vi "Track Array Replace.vi"(8 "连接端":enum16{"无连接", "前端", "后端", "前后端"}(ring), 9 "num":i32=1, 11 "output array":string[][](array[string])) -> (3 "output array 2":string[][](array[string]))   [LabVIEW 2015]
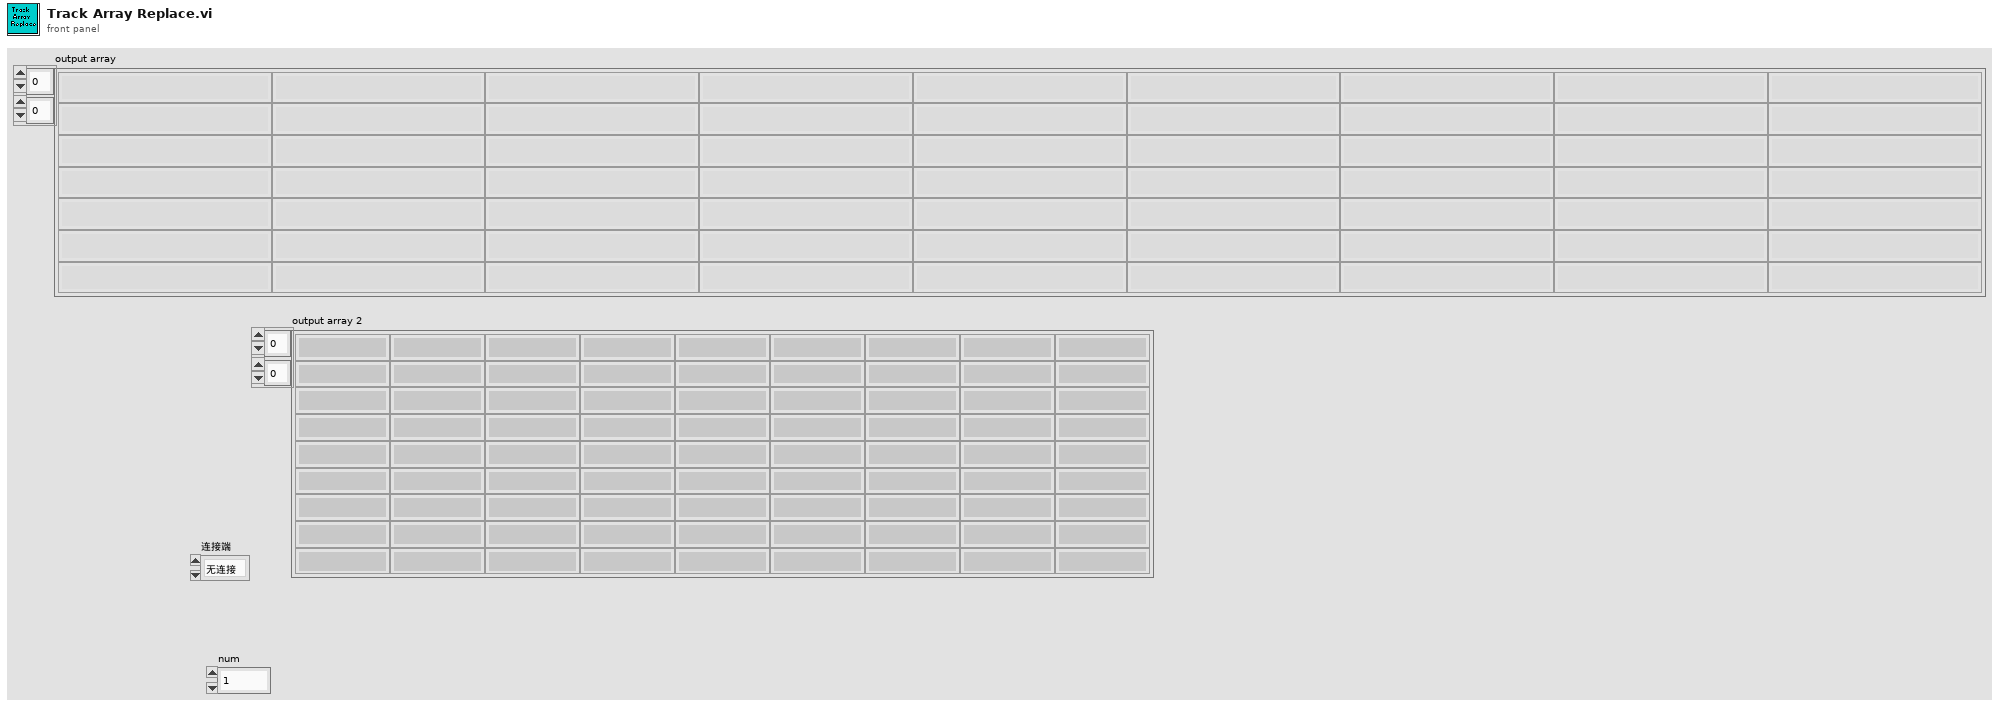
[diagram p1: front panel]
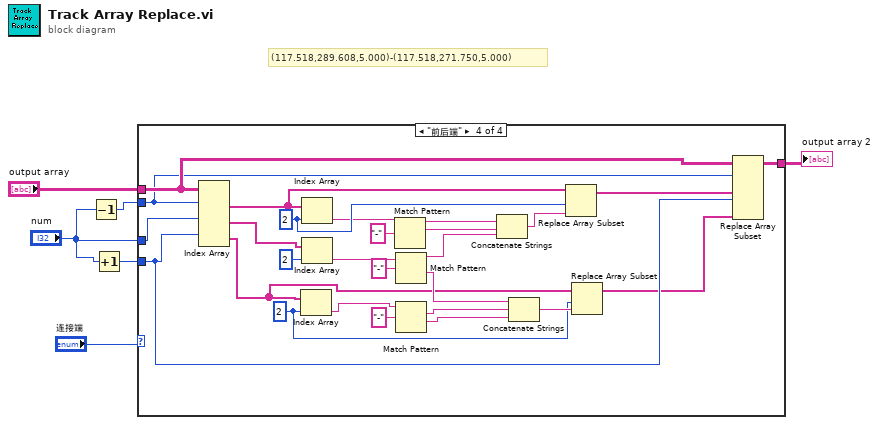
[diagram p0: block diagram]
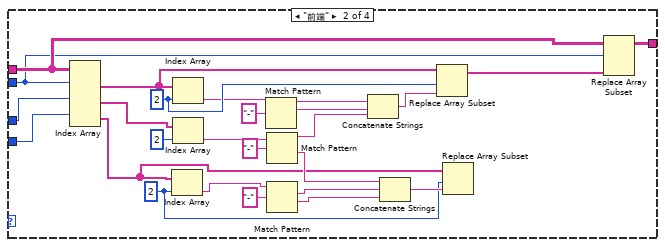
[diagram p3: hidden frame]
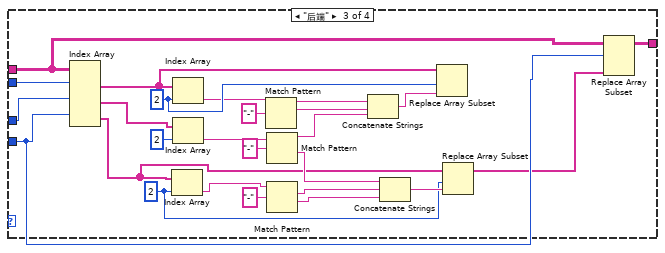
[diagram p4: hidden frame]
diagram:
  # "(117.518,289.608,5.000)-(117.518,271.750,5.000)"
  n1 = Decrement(x="num") -> (x-1=w4:i32)
  n2 = Increment(x="num") -> (x+1=w3:i32)
  n3 = case shown="\"前后端\"" "连接端" {
    tunnel: "num" -> [_ w33 w59 w86]
    tunnel: "output array" -> [w7 w12 w38 w65]
    tunnel: w4 -> [_ w11 w37 w64]
    tunnel: w3 -> [_ w9 w35 w62]
    tunnel: [w7 w8 w36 w60] -> w2
    frame "无连接", Default {
    }
    frame "前端" {
      w13 = 2 ("index")
      w28 = 2 ("index")
      n4 = Index Array(array=w12, index (row) #1=w11, index (row) #2=w33, index (row) #3=w9) -> (element #1=w27:string[], element #2=w31:string[], element #3=w15:string[])  [unwired: 3 in]
      n5 = Index Array(array=w15, index=w13) -> (element=w17:string)
      n6 = Index Array(array=w27, index=w28) -> (element=w25:string)
      n7 = Index Array(array=w31, index=2) -> (element=w30:string)
      n8 = Match Pattern(string=w25, regular expression="-") -> (before substring=w24:string, match substring=w23:string)  [unwired: 1 in, 2 out]
      n9 = Match Pattern(string=w30, regular expression="-") -> (before substring=w22:string, after substring=w19:string)  [unwired: 1 in, 2 out]
      n10 = Match Pattern(string=w17, regular expression="-") -> (match substring=w18:string, after substring=w16:string)  [unwired: 1 in, 2 out]
      n11 = Concatenate Strings(w24, w23, w22) -> (w21:string)
      n12 = Concatenate Strings(w19, w18, w16) -> (w14:string)
      n13 = Replace Array Subset(array=w27, new element=w21, index=w28) -> (w10:string[])
      n14 = Replace Array Subset(array=w15, new element=w14, index=w13) -> ()  [unwired: 1 out]
      n15 = Replace Array Subset(array=w12, new element=w10, index (row)=w11) -> (w8:string[][])  [unwired: 1 in]
    }
    frame "后端" {
      w39 = 2 ("index")
      w54 = 2 ("index")
      n16 = Index Array(array=w38, index (row) #1=w37, index (row) #2=w59, index (row) #3=w35) -> (element #1=w53:string[], element #2=w57:string[], element #3=w41:string[])  [unwired: 3 in]
      n17 = Index Array(array=w41, index=w39) -> (element=w43:string)
      n18 = Index Array(array=w53, index=w54) -> (element=w51:string)
      n19 = Index Array(array=w57, index=2) -> (element=w56:string)
      n20 = Match Pattern(string=w51, regular expression="-") -> (before substring=w50:string, match substring=w49:string)  [unwired: 1 in, 2 out]
      n21 = Match Pattern(string=w56, regular expression="-") -> (before substring=w48:string, after substring=w45:string)  [unwired: 1 in, 2 out]
      n22 = Match Pattern(string=w43, regular expression="-") -> (match substring=w44:string, after substring=w42:string)  [unwired: 1 in, 2 out]
      n23 = Concatenate Strings(w50, w49, w48) -> (w47:string)
      n24 = Concatenate Strings(w45, w44, w42) -> (w40:string)
      n25 = Replace Array Subset(array=w53, new element=w47, index=w54) -> ()  [unwired: 1 out]
      n26 = Replace Array Subset(array=w41, new element=w40, index=w39) -> (w34:string[])
      n27 = Replace Array Subset(array=w38, new element=w34, index (row)=w35) -> (w36:string[][])  [unwired: 1 in]
    }
    frame "前后端" {
      w66 = 2 ("index")
      w81 = 2 ("index")
      n28 = Index Array(array=w65, index (row) #1=w64, index (row) #2=w86, index (row) #3=w62) -> (element #1=w80:string[], element #2=w84:string[], element #3=w68:string[])  [unwired: 3 in]
      n29 = Index Array(array=w68, index=w66) -> (element=w70:string)
      n30 = Index Array(array=w80, index=w81) -> (element=w78:string)
      n31 = Index Array(array=w84, index=2) -> (element=w83:string)
      n32 = Match Pattern(string=w78, regular expression="-") -> (before substring=w77:string, match substring=w76:string)  [unwired: 1 in, 2 out]
      n33 = Match Pattern(string=w83, regular expression="-") -> (before substring=w75:string, after substring=w72:string)  [unwired: 1 in, 2 out]
      n34 = Match Pattern(string=w70, regular expression="-") -> (match substring=w71:string, after substring=w69:string)  [unwired: 1 in, 2 out]
      n35 = Concatenate Strings(w77, w76, w75) -> (w74:string)
      n36 = Concatenate Strings(w72, w71, w69) -> (w67:string)
      n37 = Replace Array Subset(array=w80, new element=w74, index=w81) -> (w63:string[])
      n38 = Replace Array Subset(array=w68, new element=w67, index=w66) -> (w61:string[])
      n39 = Replace Array Subset(array=w65, new element #1=w63, index (row) #1=w64, new element #2=w61, index (row) #2=w62) -> (w60:string[][])  [unwired: 2 in]
    }
  }
  "output array 2" <- w2
